vi "Read_parameter_string_arr.vi"(10 "Parameter name":string, 11 "String array":string[][](array[string])) -> (1 "Number of lines/number of params":i32[](array[numeric]), 2 "Parameter value":dbl, 3 "All parameter values in line":sgl[](array[numeric]), 5 "Line number":i32)   [LabVIEW 2012]
panel:
  in  "Match case?":bool
  out "Found in more than one line":bool
  out "No param name found":bool
  out "Number of lines where parameter name ofund":i32
  out "Lines and params number found":i32[][](array[numeric])
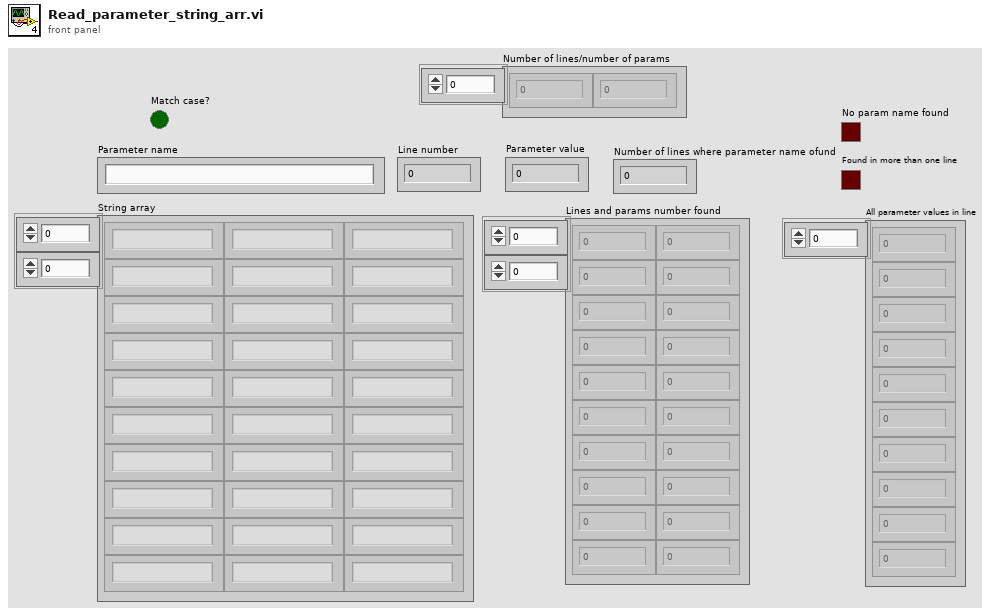
[diagram p1: front panel]
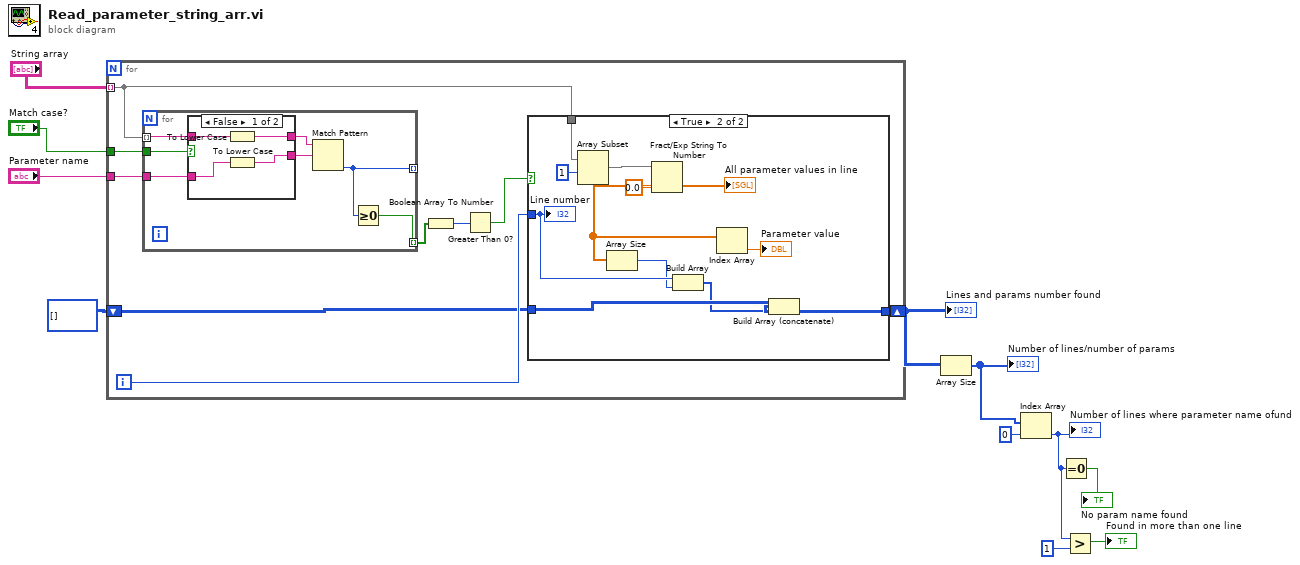
[diagram p0: block diagram]
diagram:
  n1 = for {
    tunnel: "String array" -> [w17] mode=indexing
    tunnel: "Parameter name" -> [w16]
    shift-right: [w13] -> w8
    shift-left: i32[][] [] -> [w14]
    tunnel: "Match case?" -> [w12]
    i -> [w15]
    n2 = for {
      tunnel: w17 -> [w37] mode=indexing
      tunnel: [w39] -> _ mode=indexing
      tunnel: [w38] -> w20 mode=indexing
      tunnel: w16 -> [w35]
      tunnel: w12 -> [w33]
      n3 = case shown="False" w33 {
        tunnel: w37 -> [w43 w45]
        tunnel: [w42 w45] -> w36
        tunnel: w35 -> [w41 w44]
        tunnel: [w40 w44] -> w34
        frame False {
          n4 = To Lower Case(string=w43) -> (all lower case string=w42:string)
          n5 = To Lower Case(string=w41) -> (all lower case string=w40:string)
        }
        frame True {
        }
      }
      n6 = Match Pattern(string=w36, regular expression=w34) -> (offset past match=w39:i32)  [unwired: 1 in, 3 out]
      n7 = Greater Or Equal To 0?(x=w39) -> (x >= 0?=w38:bool)
    }
    n8 = Boolean Array To Number(Boolean array=w20) -> (number=w19:u32)
    n9 = Greater Than 0?(x=w19) -> (x > 0?=w18:bool)
    n10 = case shown="True" w18 {
      tunnel: w17 -> [_ w30]
      tunnel: w15 -> [_ w24]
      tunnel: w14 -> [w21 w26]
      tunnel: [w21 w25] -> w13
      frame False {
      }
      frame True {
        n11 = Array Subset(array=w30, index=1) -> (w31:string[])  [unwired: 1 in]
        n12 = Fract/Exp String To Number(string=w31, default (0 dbl)=sgl 0.0 ("default (0 I32)")) -> (number=w28:sgl[])  [unwired: 2 in, 1 out]
        "All parameter values in line" <- w28
        n13 = Array Size(array=w28) -> (size(s)=w23:i32)
        n14 = Build Array(w24, w23) -> (w22:i32[])
        n15 = Index Array(array=w28) -> (element=→"Parameter value":sgl)  [unwired: 1 in]
        n16 = Build Array (concatenate)(w26, w22) -> (w25:i32[][])
        "Line number" <- w24
      }
    }
  }
  "Lines and params number found" <- w8
  n17 = Array Size(array=w8) -> (size(s)=w7:i32[])
  "Number of lines/number of params" <- w7
  n18 = Index Array(array=w7, index=0) -> (element=w4:i32)
  "Number of lines where parameter name ofund" <- w4
  n19 = Equal To 0?(x=w4) -> (x = 0?=→"No param name found":bool)
  n20 = Greater?(x=w4, y=1) -> (0:→"Found in more than one line":bool)
